vi "UDP Data Link - Driver Utilities - Tx to UDP Data.vi"(7 "Protocol Info":string, 8 "error in (no error)":errorcluster, 9 "In4Ver":string, 10 "SourceNodeName":string, 11 "Tx Data":dbl[](array[numeric])) -> (0 "error out":errorcluster, 3 "UDP Data":string)   [LabVIEW 2015, in "UDP Data Link Engine.lvlib"]
doc: "This VI converts Tx Data received from an RT FIFO from the inline VI to a UDP packet and returns the UDP packet so that it may be written over the network to the simulation machine. Protocl Info, System Definition version, and Source Node Name are all determined before the execution of this VI. This VI then extracts the Sequence Number and TimeStamp from the Tx Data, builds the appropriate packet header, and appends the Tx Channel data. All the data is flattened to string in little endian."
uses:
  UDP Data Link Engine.lvlib
  <vilib>/NI Veristand/Custom Device Tools/Custom Device Utility Library/Custom Device Utility Library.lvlib
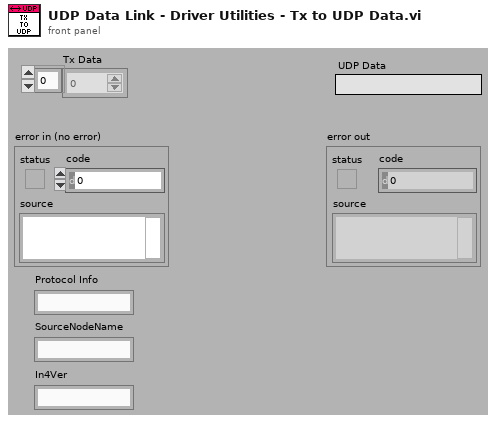
[diagram p1: front panel]
types:
  T1 = enum16{"big-endian, network order", "native, host order", "little-endian"}
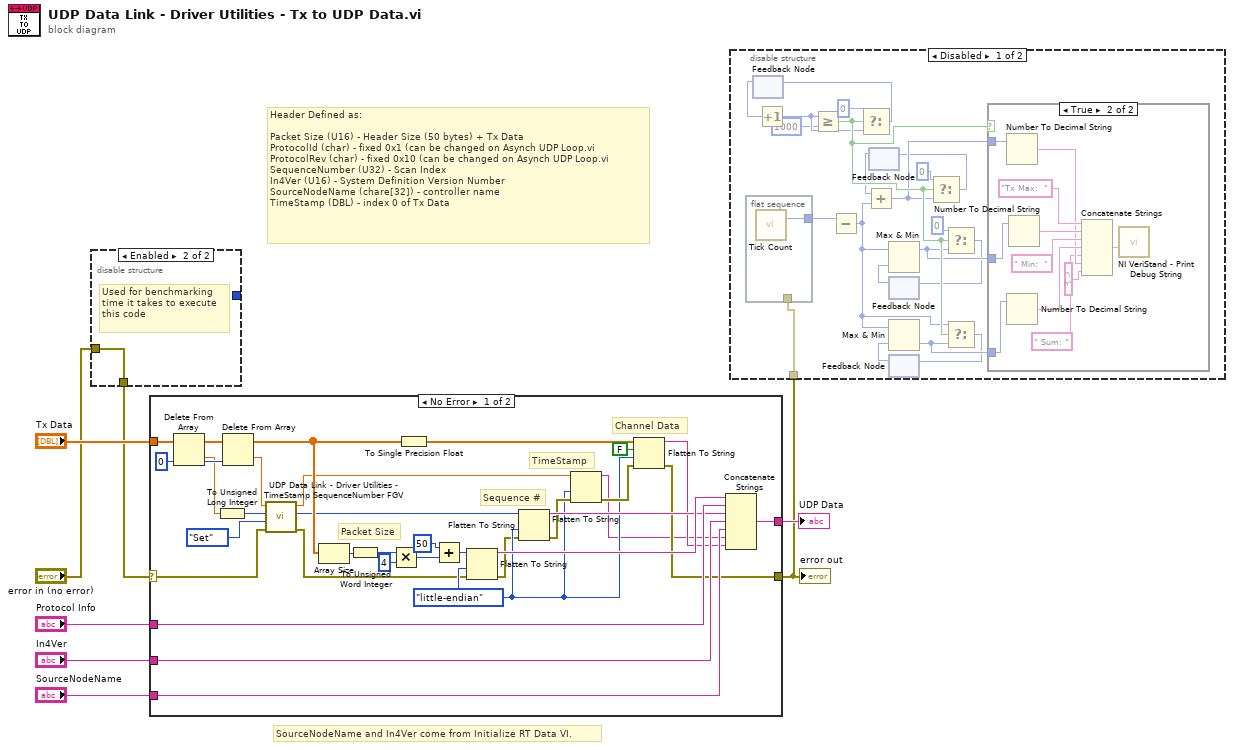
[diagram p0: block diagram]
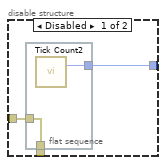
[diagram p4: hidden frame]
diagram:
  # "SourceNodeName and In4Ver come from Initialize RT Data VI."
  # "Header Defined as:\n\nPacket Size (U16) - Header Size (50 bytes) + Tx Data\nProtocolId (char) - fixed 0x1 (can be changed on Asynch UDP Loop.vi\nProtocolRev (char) - fixed 0x10 (can be changed on Asynch UDP Loop.vi\nSequenceNumber (U32) - Scan Index\nIn4Ver (U16) - System Definition Version Number\nSourceNodeName (chare[32]) - controller name\nTimeStamp (DBL) - index 0 of Tx Data"
  n1 = disable-structure shown="Enabled" {
    disable-tunnel: "error in (no error)" -> [w11 w14]
    disable-tunnel: [w10 w14] -> w1
    disable-tunnel: [w9 _] -> _
    frame Disabled {
      n2 = flat-sequence {
        tunnel: [w13] -> w9
        tunnel: w11 -> [w12]
        tunnel: [w12] -> w10
        frame #0 {
          n3 = call "Tick Count2"() -> ("Tick Count(uSec)"=w13:u32)
        }
      }
    }
    frame Enabled {
      # "Used for benchmarking time it takes to execute this code"
    }
  }
  n4 = case shown="No Error" w1 {
    selector: w1 -> [w19 w48]
    tunnel: "Tx Data" -> [w42 _]
    tunnel: "Protocol Info" -> [w38 _]
    tunnel: [w30 w48] -> w3
    tunnel: "In4Ver" -> [w36 _]
    tunnel: "SourceNodeName" -> [w35 _]
    tunnel: [w31 _] -> w4
    frame No Error {
      w32 = T1."little-endian" ("byte order (0:big-endian, network order)")
      w25 = 0 ("index")
      # "Packet Size"
      # "TimeStamp"
      # "Channel Data"
      # "Sequence #"
      n5 = Delete From Array(array=w42, index=w25) -> (deleted portion=w24:dbl, array with subset deleted=w26:dbl[])  [unwired: 1 in]
      n6 = To Unsigned Long Integer(number=w24) -> (unsigned 32bit integer=w21:u32)
      n7 = Delete From Array(array=w26, index=w25) -> (deleted portion=w16:dbl, array with subset deleted=w23:dbl[])  [unwired: 1 in]
      n8 = call "UDP Data Link - Driver Utilities - TimeStamp SequenceNumber FGV.vi"("error in (no error)"=w19, "Enum"=enum16{"Get", "Set"}."Set", "Sequence Number In"=w21, "Timestamp In"=w16) -> ("error out"=w18:errorcluster, "Sequence Number Out"=w20:u32, "Timestamp Out"=w15:dbl)  [unwired: 5 in]
      n9 = Array Size(array=w23) -> (size(s)=w47:i32)
      n10 = To Unsigned Word Integer(number=w47) -> (unsigned 16bit integer=w43:u16)
      n11 = Multiply(x=w43, y=u16 4) -> (x*y=w45:u16)
      n12 = To Single Precision Float(number=w23) -> (single precision float=w29:sgl[])
      n13 = Add(x=u16 50, y=w45) -> (x+y=w40:u16)
      n14 = Flatten To String(anything=w40, byte order (0:big-endian, network order)=w32, error in (no error)=w18) -> (data string=w39:string, error out=w17:errorcluster)  [unwired: 1 in, 1 out]
      n15 = Flatten To String(anything=w20, byte order (0:big-endian, network order)=w32, error in (no error)=w17) -> (data string=w37:string, error out=w34:errorcluster)  [unwired: 1 in, 1 out]
      n16 = Flatten To String(anything=w15, byte order (0:big-endian, network order)=w32, error in (no error)=w34) -> (data string=w27:string, error out=w33:errorcluster)  [unwired: 1 in, 1 out]
      n17 = Flatten To String(anything=w29, prepend array or string size? (T)=FALSE, byte order (0:big-endian, network order)=w32, error in (no error)=w33) -> (data string=w28:string, error out=w30:errorcluster)  [unwired: 1 out]
      n18 = Concatenate Strings(w39, w38, w37, w36, w35, w27, w28) -> (w31:string)
    }
    frame Error {
    }
  }
  "UDP Data" <- w4
  "error out" <- w3
  n19 = disable-structure shown="Disabled" {
    disable-tunnel: w3 -> [w50 _]
    frame Disabled {
      n20 = flat-sequence {
        tunnel: [w81] -> w51
        tunnel: w50 -> [_]
        frame #0 {
          n21 = call "Tick Count"() -> ("Tick Count(uSec)"=w81:u32)
        }
      }
      n22 = feedback #1() -> (w52:i32)  [unwired: 1 in]
      n23 = Increment(x=w52) -> (x+1=w56:i32)
      n24 = Greater Or Equal?(x=w56, y=1000) -> (x >= y?=w69:bool)
      n25 = Subtract(x=w51) -> (y=w49:u32, x-y=w62:u32)
      n26 = Select(t=0, s=w69, f=w56) -> (s? t:f=w54:i32)
      n27 = feedback-in #1(w54) -> ()
      n28 = feedback #2() -> (w57:u32)  [unwired: 1 in]
      n29 = Add(x=w57, y=w62) -> (x+y=w68:u32)
      n30 = feedback #3() -> (w59:u32)  [unwired: 1 in]
      n31 = Max & Min(x=w62, y=w59) -> (max(x,y)=w67:u32)  [unwired: 1 out]
      n32 = feedback #4() -> (w61:u32)  [unwired: 1 in]
      n33 = Max & Min(x=w62, y=w61) -> (min(x,y)=w66:u32)  [unwired: 1 out]
      n34 = Select(t=u32 0, s=w69, f=w68) -> (s? t:f=w65:u32)
      n35 = feedback-in #2(w65) -> ()
      n36 = Select(t=u32 0, s=w69, f=w67) -> (s? t:f=w63:u32)
      n37 = feedback-in #3(w63) -> ()
      n38 = Select(t=w62, s=w69, f=w66) -> (s? t:f=w64:u32)
      n39 = feedback-in #4(w64) -> ()
      n40 = case shown="True" w69 {
        tunnel: w66 -> [_ w73]
        tunnel: w67 -> [_ w72]
        tunnel: w68 -> [_ w71]
        frame False {
        }
        frame True {
          n41 = Number To Decimal String(number=w71) -> (decimal integer string=w75:string)  [unwired: 1 in]
          n42 = Number To Decimal String(number=w73) -> (decimal integer string=w77:string)  [unwired: 1 in]
          n43 = Number To Decimal String(number=w72) -> (decimal integer string=w80:string)  [unwired: 1 in]
          n44 = Concatenate Strings("Tx Max:  " ("string"), w80, " Min:  " ("string"), w77, " Sum: " ("string"), w75, "\n" ("string")) -> (w79:string)
          n45 = call <vilib>:"NI VeriStand - Print Debug String.vi"("Debug String"=w79) -> ()  [unwired: 9 in, 1 out]
        }
      }
    }
    frame Enabled {
      # "Used for benchmarking this code. On a 8130, it was measured to have max execution time of ~30 usec, min execution time of ~9 usec, and average execution time of ~10.1 usec. There were only 4 Tx channels being sent when making this benchmark."
    }
  }
